vi "Factory.vi"(9 "Blacklist Class":T1, 10 "VI Refnum":refnum<vi>, 11 "CLI":refnum<class "CLI.lvclass">) -> (0 "error out":errorcluster, 3 "Blacklist out":refnum<class "Blacklist.lvclass">)   [LabVIEW 2014, in "lvbuildsecurity.lvlib" / "Blacklist.lvclass"]
uses:
  Blacklist.lvclass
  ctlBlacklistClass.ctl
  <vilib>/Wiresmith Technology/LabVIEW CLI/CLI Class/CLI.lvclass
  Blacklist.lvclass/Blacklist.ctl
  lvbuildsecurity.lvlib
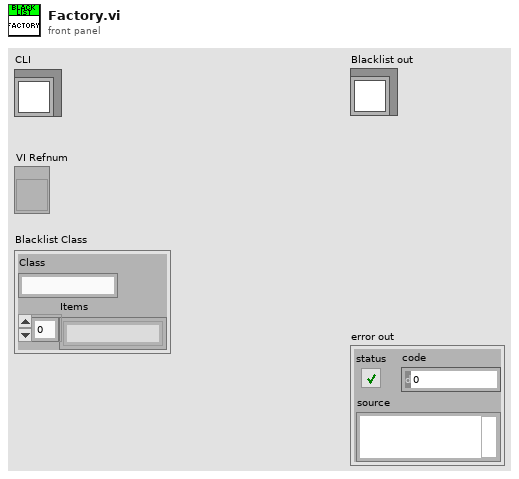
[diagram p1: front panel]
types:
  T1 = typedef "lvbuildsecurity.lvlib/ctlBlacklistClass.ctl" = cluster{"Class":string, "Items":string[]}
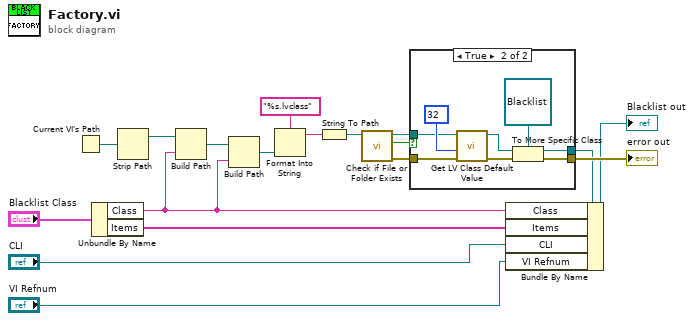
[diagram p0: block diagram]
diagram:
  n1 = Current VI's Path() -> (path=w8:path)
  n2 = Unbundle By Name("Blacklist Class") -> ("Class"=w3:string, "Items"=w5:string[])
  n3 = Strip Path(path=w8) -> (stripped path=w7:path)  [unwired: 1 out]
  n4 = Build Path(base path=w7, name or relative path=w3) -> (appended path=w10:path)
  n5 = Build Path(base path=w10, name or relative path=w3) -> (appended path=w9:path)
  n6 = Format Into String(format string="%s.lvclass", w9) -> (resulting string=w12:string)  [unwired: 2 in, 1 out]
  n7 = String To Path(string=w12) -> (path=w11:path)
  n8 = call <vilib>:"Check if File or Folder Exists.vi"("path"=w11) -> ("error out"=w16:errorcluster, "file or folder exists?"=w15:bool, "dup path"=w17:path)  [unwired: 8 in]
  n9 = case shown="True" w15 {
    tunnel: [_ w24] -> w6
    tunnel: [w19 w22] -> w18
    tunnel: w17 -> [_ w21]
    tunnel: w16 -> [w19 w20]
    frame False {
    }
    frame True {
      n10 = call <vilib>:"Get LV Class Default Value.vi"("error in (no error)"=w20, "options"=u32 32, "class path"=w21) -> ("error out"=w25:errorcluster, "object"=w26:refnum<class>)  [unwired: 7 in]
      n11 = To More Specific Class(target class=refnum<class "Blacklist.lvclass"> refnum ("lvbuildsecurity.lvlib:BlacklistProcessor.lvclass"), reference=w26, error in=w25) -> (specific class reference=w24:refnum<class "Blacklist.lvclass">, error out=w22:errorcluster)
    }
  }
  "error out" <- w18
  n12 = Bundle By Name(cluster=w6, "Class"=w3, "Items"=w5, "CLI"="CLI", "VI Refnum"="VI Refnum") -> (→"Blacklist out":refnum<class "Blacklist.lvclass">)
